vi "associateToLandmark.vi"(9 "noFoundLandmarks":i32, 10 "foundLandmarks":T1, 11 "currentLandmark":dbl[](array[numeric])) -> (3 "associatedFoundLandmark":i32)   [LabVIEW 2009, in "LV_SLAM.lvlib"]
uses:
  LV_SLAM.lvlib
  <vilib>/Analysis/Matrix/Datatypes/RealMatrix.ctl
  <vilib>/Analysis/Matrix/NI_Matrix.lvlib
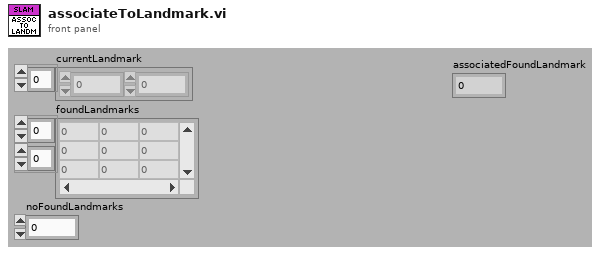
[diagram p1: front panel]
types:
  T1 = typedef "NI_Matrix.lvlib/RealMatrix.ctl" = dbl[][]
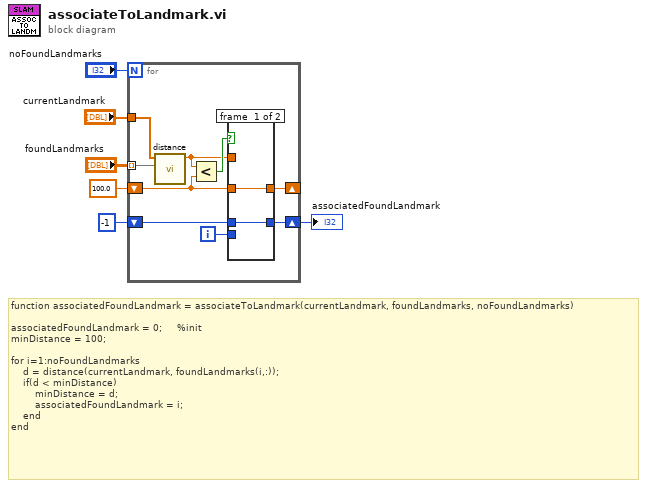
[diagram p0: block diagram]
diagram:
  # "function associatedFoundLandmark = associateToLandmark(currentLandmark, foundLandmarks, noFoundLandmarks)\n\nassociatedFoundLandmark = 0;     %init\nminDistance = 100;\n\nfor i=1:noFoundLandmarks\n    d = distance(currentLandmark, foundLandmarks(i,:));\n    if(d < minDistance)\n        minDistance = d;\n        associatedFoundLandmark = i;\n    end\nend"
  n1 = for {
    N: "noFoundLandmarks" -> [_]
    tunnel: "currentLandmark" -> [w15]
    tunnel: "foundLandmarks" -> [w14] mode=indexing
    shift-right: [w7] -> _
    shift-left: 100.0 ("noFoundLandmarks") -> [w11]
    shift-right: [w8] -> w1
    shift-left: -1 ("associatedFoundLandmark") -> [w10]
    i -> [w9]
    n2 = call "distance.vi"("X2"=w14, "X1"=w15) -> ("d"=w12:dbl)  [unwired: 9 in]
    n3 = Less?(x=w12, y=w11) -> (x < y?=w13:bool)
    n4 = case shown="False" w13 {
      tunnel: w12 -> [_ w18]
      tunnel: w11 -> [w16 _]
      tunnel: w10 -> [w17 _]
      tunnel: w9 -> [_ w19]
      tunnel: [w17 w19] -> w8
      tunnel: [w16 w18] -> w7
      frame #0 {
      }
      frame #1 {
      }
    }
  }
  "associatedFoundLandmark" <- w1
